vi "create messages summary.vi"(1 "messages map":map{u32, T1}(c390)) -> (0 "messages summary":string)   [LabVIEW 2024, in "atsj peakcan basic.lvlib"]
uses:
  atsj peakcan basic.lvlib
  message type.ctl
  message.ctl
  message with stats.ctl
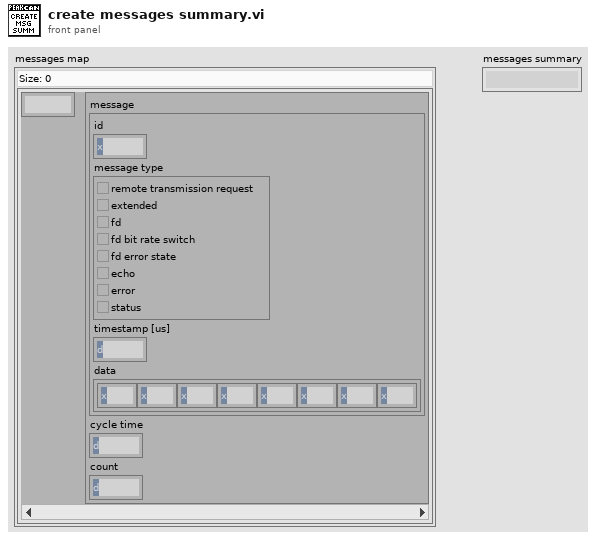
[diagram p1: front panel]
types:
  T1 = typedef "atsj peakcan basic.lvlib/message with stats.ctl" = cluster{"message":T2, "cycle time":u64, "count":u64}
  T2 = typedef "atsj peakcan basic.lvlib/message.ctl" = cluster{"id":u32, "message type":T3, "timestamp [us]":u64, "data":u8[]}
  T3 = typedef "atsj peakcan basic.lvlib/message type.ctl" = cluster{"remote transmission request ":bool, "extended":bool, "fd":bool, "fd bit rate switch":bool, "fd error state":bool, "echo":bool, "error":bool, "status":bool}
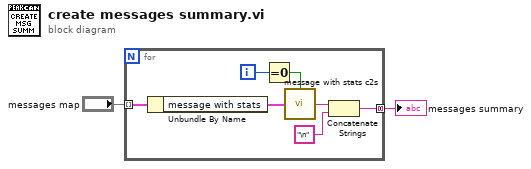
[diagram p0: block diagram]
diagram:
  n1 = for {
    tunnel: "messages map" -> [w4] mode=indexing
    tunnel: [w9] -> w1 mode=concatenating
    i -> [w6]
    n2 = Unbundle By Name(w4) -> ("message with stats"=w3:T1)
    n3 = Equal To 0?(x=w6) -> (x = 0?=w5:bool)
    n4 = call "message with stats c2s.vi"("cluster"=w3, "add header? (F)"=w5) -> ("string"=w7:string)
    n5 = Concatenate Strings(w7, "\n") -> (w9:string)
  }
  "messages summary" <- w1
